vi "Write Analogue.vi"(8 "error in (no error)":errorcluster, 9 "Output":bool, 10 "Channel index(0)":i32, 11 "niPower in":refnum<class "NI DC Power.lvclass">) -> (0 "error out":errorcluster, 2 "Success?":bool, 3 "niPower out":refnum<class "NI DC Power.lvclass">)   [LabVIEW 2025, in "Power Supply.lvlib" / "NI DC Power.lvclass"]
uses:
  NI DC Power.lvclass
  NI DC Power.lvclass/NI DC Power.ctl
  b5821778-c9e7-4ba9-a9c1-1b7d3418e9a7.vi
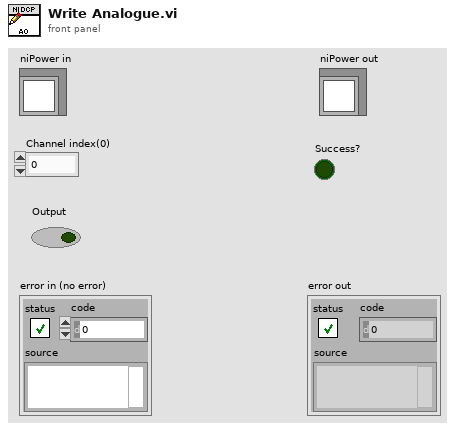
[diagram p1: front panel]
types:
  T1 = typedef "Abstract Engine.lvlibp/Abstract Instrument.lvclass/Channel.ctl" = cluster{"Alias":string, "DataType":enum16{"Anaolg Input", "Waveform"}, "Unit":enum16{"---", "V", "A", "Ohm", "Hz", "uF", "degC", "deg"}, "Upper limit":dbl, "Lower limit":dbl, "Measurement":variant}
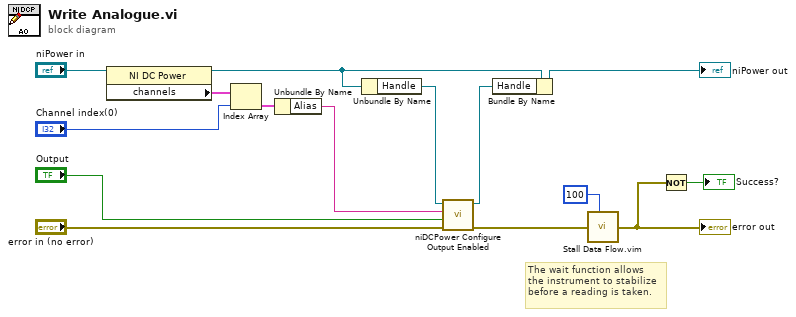
[diagram p0: block diagram]
diagram:
  # "The wait function allows \nthe instrument to stabilize\nbefore a reading is taken."
  n1 = property class="NI DC Power"(reference="niPower in") -> (reference out=w1:refnum<class "NI DC Power.lvclass">, "channels"=w4:T1[])  [unwired: 1 in, 1 out]
  n2 = Index Array(array=w4, index="Channel index(0)") -> (element=w3:T1)
  n3 = Unbundle By Name(w3) -> ("Alias"=w2:string)
  n4 = Unbundle By Name(w1) -> ("Handle"=w12:refnum<k15>)
  n5 = call <instrlib>:"niDCPower Configure Output Enabled.vi"("error in (no error)"="error in (no error)", "output enabled"="Output", "channel name"=w2, "instrument handle"=w12) -> ("error out"=w11:errorcluster, "instrument handle out"=w5:refnum<k15>)  [unwired: 6 in]
  n6 = Bundle By Name(cluster=w1, "Handle"=w5) -> (→"niPower out":refnum<class "NI DC Power.lvclass">)
  n7 = call "Stall Data Flow.vim"("value in"=w11, "milliseconds to wait"=u32 100 ("millisecond timer value")) -> ("value out"=w9:errorcluster)  [unwired: 1 out]
  "error out" <- w9
  n8 = Not(x=w9) -> (.not. x?=→"Success?":bool)
